vi "TcpipCmdVerify.vi"(5 "CMDrx":string) -> (2 "QueneElement":cluster{"TCPIP CMD":T1, variant})   [LabVIEW 2024]
uses:
  Control/TCPIP CMD.ctl
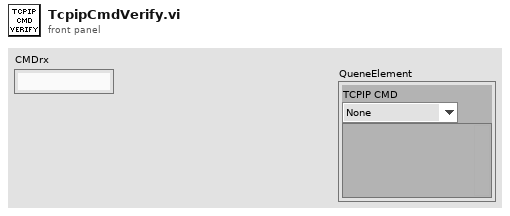
[diagram p1: front panel]
types:
  T1 = typedef "TCPIP CMD.ctl" = enum16{"None", "REMOTE", "LOCAL", "ERES", "ERROR?", "SERVO", "SERVO?", "DIRN", "DIRN?", "TESTMODE", "TESTMODE?", "SPEED", "SPEED?", "TORQUE", "TORQUE?", "POSITION", "POSRES", "TPS", "TPS?", "PS", "PS?", "PSON", "PSOFF", "COLUMNS", "DATA", "RAMP", "STOP", "DISCONN", "STARTLOG", "STOPLOG"}
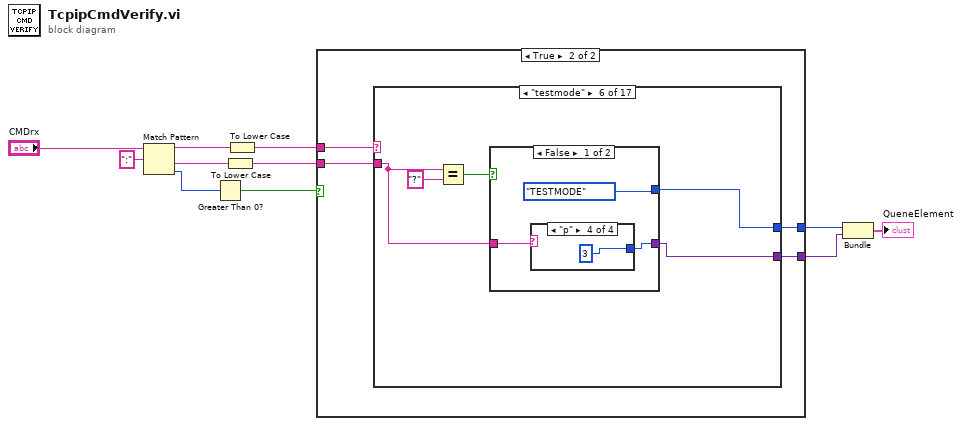
[diagram p0: block diagram]
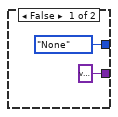
[diagram p2: hidden frame]
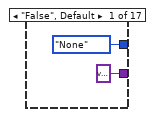
[diagram p3: hidden frame]
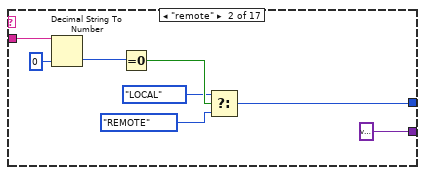
[diagram p4: hidden frame]
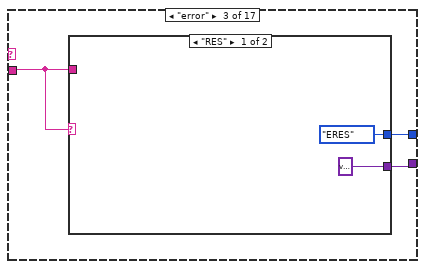
[diagram p5: hidden frame]
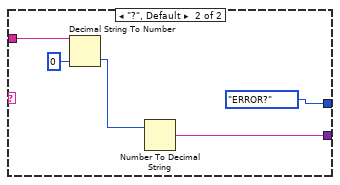
[diagram p6: hidden frame]
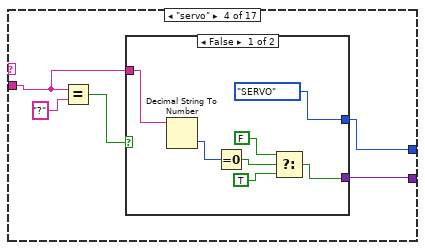
[diagram p7: hidden frame]
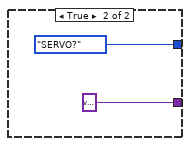
[diagram p8: hidden frame]
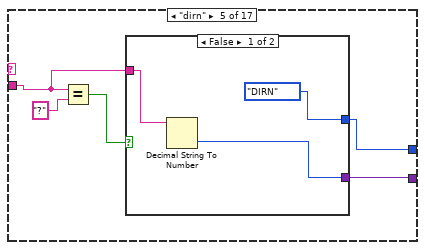
[diagram p9: hidden frame]
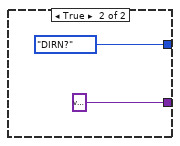
[diagram p10: hidden frame]
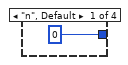
[diagram p11: hidden frame]
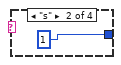
[diagram p12: hidden frame]
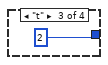
[diagram p13: hidden frame]
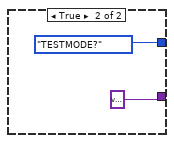
[diagram p14: hidden frame]
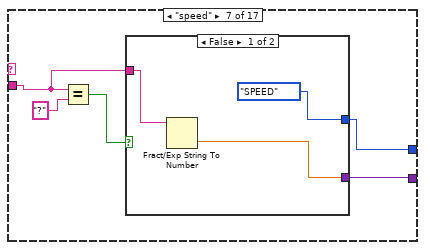
[diagram p15: hidden frame]
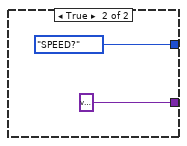
[diagram p16: hidden frame]
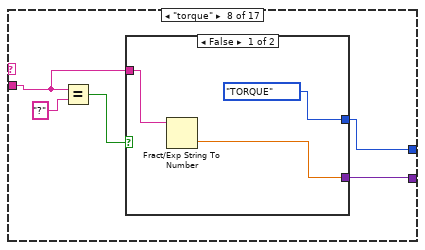
[diagram p17: hidden frame]
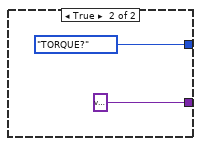
[diagram p18: hidden frame]
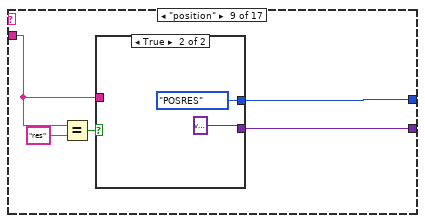
[diagram p19: hidden frame]
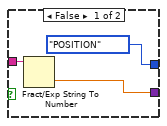
[diagram p20: hidden frame]
diagram:
  n1 = Match Pattern(string="CMDrx", regular expression=":") -> (before substring=w7:string, after substring=w5:string, offset past match=w9:i32)  [unwired: 1 in, 1 out]
  n2 = Greater Than 0?(x=w9) -> (x > 0?=w8:bool)
  n3 = To Lower Case(string=w5) -> (all lower case string=w1:string)
  n4 = To Lower Case(string=w7) -> (all lower case string=w6:string)
  n5 = case shown="True" w8 {
    tunnel: w6 -> [_ w17]
    tunnel: w1 -> [_ w16]
    tunnel: [TCPIP_CMD."None" ("TCPIP CMD") w15] -> w4
    tunnel: [variant w14] -> w3
    frame False {
    }
    frame True {
      n6 = case shown="\"testmode\"" w17 {
        tunnel: w16 -> [_ w27 w28 w40 w54 w64 w78 w88 w99 w108 w116 w144 w152 _ _ w167 _]
        tunnel: [TCPIP_CMD."None" ("TCPIP CMD") w23 w29 w39 w53 w63 w77 w87 w96 w107 w118 w139 w145 TCPIP_CMD."STOP" ("TCPIP CMD") TCPIP_CMD."DISCONN" ("TCPIP CMD") TCPIP_CMD."STARTLOG" ("TCPIP CMD") TCPIP_CMD."STOPLOG" ("TCPIP CMD")] -> w15
        tunnel: [variant variant w30 w38 w52 w62 w76 w86 w100 w106 w117 variant w146 variant variant w165 variant] -> w14
        frame "False", Default {
        }
        frame "remote" {
          n7 = Decimal String To Number(string=w27, default (0L)=0 ("default (0 I32)")) -> (number=w25:i32)  [unwired: 1 in, 1 out]
          n8 = Equal To 0?(x=w25) -> (x = 0?=w24:bool)
          n9 = Select(t=TCPIP_CMD."LOCAL" ("TCPIP CMD"), s=w24, f=TCPIP_CMD."REMOTE" ("TCPIP CMD")) -> (s? t:f=w23:T1)
        }
        frame "error" {
          n10 = case shown="\"RES\"" w28 {
            tunnel: w28 -> [_ w36]
            tunnel: [variant w34] -> w30
            tunnel: [TCPIP_CMD."ERES" ("TCPIP CMD") TCPIP_CMD."ERROR?" ("TCPIP CMD")] -> w29
            frame "RES" {
            }
            frame "?", Default {
              n11 = Decimal String To Number(string=w36, default (0L)=0 ("default (0 I32)")) -> (number=w35:i32)  [unwired: 1 in, 1 out]
              n12 = Number To Decimal String(number=w35) -> (decimal integer string=w34:string)  [unwired: 1 in]
            }
          }
        }
        frame "servo" {
          n13 = Equal?(x=w40, y="?") -> (x = y?=w41:bool)
          n14 = case shown="False" w41 {
            tunnel: w40 -> [w48 _]
            tunnel: [TCPIP_CMD."SERVO" ("TCPIP CMD") TCPIP_CMD."SERVO?" ("TCPIP CMD")] -> w39
            tunnel: [w43 variant] -> w38
            frame False {
              n15 = Decimal String To Number(string=w48) -> (number=w47:i32)  [unwired: 2 in, 1 out]
              n16 = Equal To 0?(x=w47) -> (x = 0?=w46:bool)
              n17 = Select(t=FALSE, s=w46, f=TRUE) -> (s? t:f=w43:bool)
            }
            frame True {
            }
          }
        }
        frame "dirn" {
          n18 = Equal?(x=w54, y="?") -> (x = y?=w55:bool)
          n19 = case shown="False" w55 {
            tunnel: w54 -> [w58 _]
            tunnel: [TCPIP_CMD."DIRN" ("TCPIP CMD") TCPIP_CMD."DIRN?" ("TCPIP CMD")] -> w53
            tunnel: [w57 variant] -> w52
            frame False {
              n20 = Decimal String To Number(string=w58) -> (number=w57:i32)  [unwired: 2 in, 1 out]
            }
            frame True {
            }
          }
        }
        frame "testmode" {
          n21 = Equal?(x=w64, y="?") -> (x = y?=w65:bool)
          n22 = case shown="False" w65 {
            tunnel: [TCPIP_CMD."TESTMODE" ("TCPIP CMD") TCPIP_CMD."TESTMODE?" ("TCPIP CMD")] -> w63
            tunnel: w64 -> [w68 _]
            tunnel: [w67 variant] -> w62
            frame False {
              n23 = case shown="\"p\"" w68 {
                tunnel: [u16 0 u16 1 u16 2 u16 3] -> w67
                frame "n", Default {
                }
                frame "s" {
                }
                frame "t" {
                }
                frame "p" {
                }
              }
            }
            frame True {
            }
          }
        }
        frame "speed" {
          n24 = Equal?(x=w78, y="?") -> (x = y?=w79:bool)
          n25 = case shown="False" w79 {
            tunnel: w78 -> [w82 _]
            tunnel: [TCPIP_CMD."SPEED" ("TCPIP CMD") TCPIP_CMD."SPEED?" ("TCPIP CMD")] -> w77
            tunnel: [w81 variant] -> w76
            frame False {
              n26 = Fract/Exp String To Number(string=w82) -> (number=w81:dbl)  [unwired: 3 in, 1 out]
            }
            frame True {
            }
          }
        }
        frame "torque" {
          n27 = Equal?(x=w88, y="?") -> (x = y?=w89:bool)
          n28 = case shown="False" w89 {
            tunnel: w88 -> [w92 _]
            tunnel: [TCPIP_CMD."TORQUE" ("TCPIP CMD") TCPIP_CMD."TORQUE?" ("TCPIP CMD")] -> w87
            tunnel: [w91 variant] -> w86
            frame False {
              n29 = Fract/Exp String To Number(string=w92) -> (number=w91:dbl)  [unwired: 3 in, 1 out]
            }
            frame True {
            }
          }
        }
        frame "position" {
          n30 = Equal?(x=w99, y="res") -> (x = y?=w97:bool)
          n31 = case shown="True" w97 {
            tunnel: [w103 variant] -> w100
            tunnel: w99 -> [w102 _]
            tunnel: [TCPIP_CMD."POSITION" ("TCPIP CMD") TCPIP_CMD."POSRES" ("TCPIP CMD")] -> w96
            frame False {
              n32 = Fract/Exp String To Number(string=w102) -> (number=w103:dbl)  [unwired: 3 in, 1 out]
            }
            frame True {
            }
          }
        }
        frame "tps" {
          n33 = Equal?(x=w108, y="?") -> (x = y?=w109:bool)
          n34 = case shown="False" w109 {
            tunnel: w108 -> [w112 _]
            tunnel: [TCPIP_CMD."TPS" ("TCPIP CMD") TCPIP_CMD."TPS?" ("TCPIP CMD")] -> w107
            tunnel: [w111 variant] -> w106
            frame False {
              n35 = Fract/Exp String To Number(string=w112) -> (number=w111:dbl)  [unwired: 3 in, 1 out]
            }
            frame True {
            }
          }
        }
        frame "ps" {
          (unwired) "?" ("y")
          n36 = case shown="\"?\"" w116 {
            tunnel: w116 -> [w120 _ _ _]
            tunnel: [TCPIP_CMD."PS" ("TCPIP CMD") TCPIP_CMD."PS?" ("TCPIP CMD") TCPIP_CMD."PSON" ("TCPIP CMD") TCPIP_CMD."PSOFF" ("TCPIP CMD")] -> w118
            tunnel: [w128 variant variant variant] -> w117
            frame "False", Default {
              n37 = Spreadsheet String To Array(delimiter (Tab)="|" ("regular expression"), format string="%s", spreadsheet string=w120, array type (2D Dbl)=string[] []) -> (array=w125:string[])
              n38 = Index Array(array=w125) -> (element #1=w124:string, element #2=w123:string, element #3=w122:string)  [unwired: 3 in]
              n39 = Fract/Exp String To Number(string=w124) -> (number=w130:dbl)  [unwired: 3 in, 1 out]
              n40 = Fract/Exp String To Number(string=w123) -> (number=w129:dbl)  [unwired: 3 in, 1 out]
              n41 = Fract/Exp String To Number(string=w122) -> (number=w121:dbl)  [unwired: 3 in, 1 out]
              n42 = Bundle(w130, w129, w121) -> (w128:cluster{dbl, dbl, dbl})  [unwired: 1 in]
            }
            frame "?" {
            }
            frame "on" {
            }
            frame "off" {
            }
          }
        }
        frame "meas" {
          n43 = Equal?(x=w144, y="data") -> (x = y?=w142:bool)
          n44 = Select(t=TCPIP_CMD."DATA" ("TCPIP CMD"), s=w142, f=TCPIP_CMD."COLUMNS" ("TCPIP CMD")) -> (s? t:f=w139:T1)
        }
        frame "ramp" {
          n45 = Match Pattern(string=w152, regular expression="|") -> (before substring=w148:string, after substring=w147:string, offset past match=w150:i32)  [unwired: 1 in, 1 out]
          n46 = Greater Or Equal To 0?(x=w150) -> (x >= 0?=w149:bool)
          n47 = case shown="True" w149 {
            tunnel: w148 -> [_ w160]
            tunnel: w147 -> [_ w159]
            tunnel: [variant w156] -> w146
            tunnel: [TCPIP_CMD."None" ("TCPIP CMD") TCPIP_CMD."RAMP" ("TCPIP CMD")] -> w145
            frame False {
            }
            frame True {
              n48 = Fract/Exp String To Number(string=w160) -> (number=w158:dbl)  [unwired: 3 in, 1 out]
              n49 = Fract/Exp String To Number(string=w159) -> (number=w157:dbl)  [unwired: 3 in, 1 out]
              n50 = Bundle(w158, w157) -> (w156:cluster{dbl, dbl})  [unwired: 1 in]
            }
          }
        }
        frame "stoptest" {
        }
        frame "disconn" {
        }
        frame "startlog" {
          n51 = Fract/Exp String To Number(string=w167, default (0 dbl)=0.0 ("default (0 DBL)")) -> (number=w165:dbl)  [unwired: 2 in, 1 out]
        }
        frame "stoplog" {
        }
      }
    }
  }
  n52 = Bundle("TCPIP CMD"=w4, w3) -> (→"QueneElement":cluster{"TCPIP CMD":T1, variant})  [unwired: 1 in]
